vi "RT_Aerodynamic_Force_in_DLR_Navigation_Reference_System_2 (SubVI).vi"(0 "Data":dbl[][](array[numeric]), 2 "input cluster 3":T4, 5 "i":i32, 7 "output cluster":T3, 9 "Rotation":T1, 11 "Vehicle Parameters":T2) -> (4 "FA":dbl[](array[numeric]), 15 "FA_b":dbl[](array[numeric]))   [LabVIEW 2017]
uses:
  <vilib>/Analysis/coordinate.llb/Euler Rotation Order.ctl
  <vilib>/Analysis/baseanly.llb/Real A x B.vi
  <vilib>/Analysis/Matrix/Numeric/Conversions/Array To Matrix - RA.vi
  <vilib>/Analysis/Matrix/Numeric/Conversions/Array To Matrix - RA2.vi
  <vilib>/Analysis/Matrix/Numeric/Conversions/Matrix To Array - RM.vi
  <vilib>/Analysis/NI_AALPro.lvlib
  <vilib>/Analysis/Matrix/NI_Matrix.lvlib
  <vilib>/Analysis/NI_AALBase.lvlib
panel:
  out "FAl":dbl[](array[numeric])
  out "FAy":dbl[](array[numeric])
  out "FAp":dbl[](array[numeric])
  out "FA_long":dbl
  out "FA_yaw":dbl
  out "FA_pitch":dbl
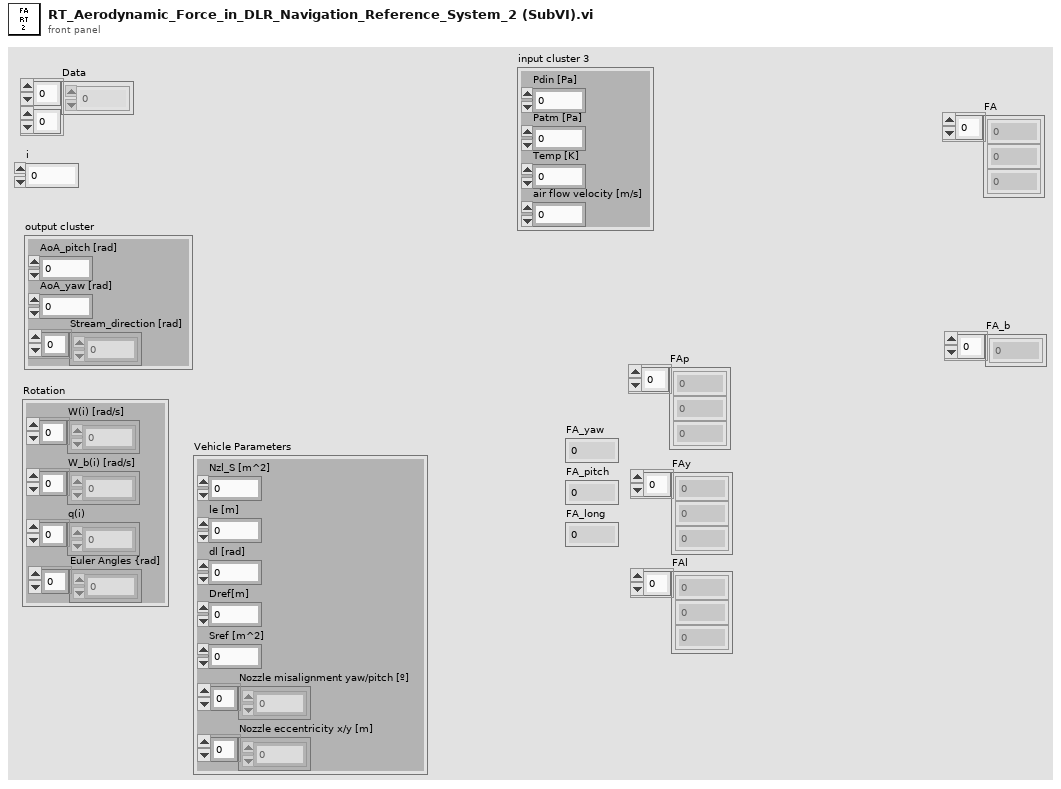
[diagram p1: front panel]
types:
  T1 = cluster{"W(i) [rad/s]":dbl[], "W_b(i) [rad/s]":dbl[], "q(i)":dbl[], "Euler Angles {rad]":dbl[]}
  T2 = cluster{"Nzl_S [m^2]":dbl, "le [m]":dbl, "dl [rad]":dbl, "Dref[m]":dbl, "Sref [m^2]":dbl, "Nozzle misalignment yaw/pitch [º]":dbl[], "Nozzle eccentricity x/y [m]":dbl[]}
  T3 = cluster{"AoA_pitch [rad]":dbl, "AoA_yaw [rad]":dbl, "Stream_direction [rad]":dbl[]}
  T4 = cluster{"Pdin [Pa]":dbl, "Patm [Pa]":dbl, "Temp [K]":dbl, "air flow velocity [m/s]":dbl}
  T5 = typedef "NI_AALPro.lvlib/Euler Rotation Order.ctl" = u16
  T6 = typedef "NI_Matrix.lvlib/RealMatrix.ctl" = dbl[][]
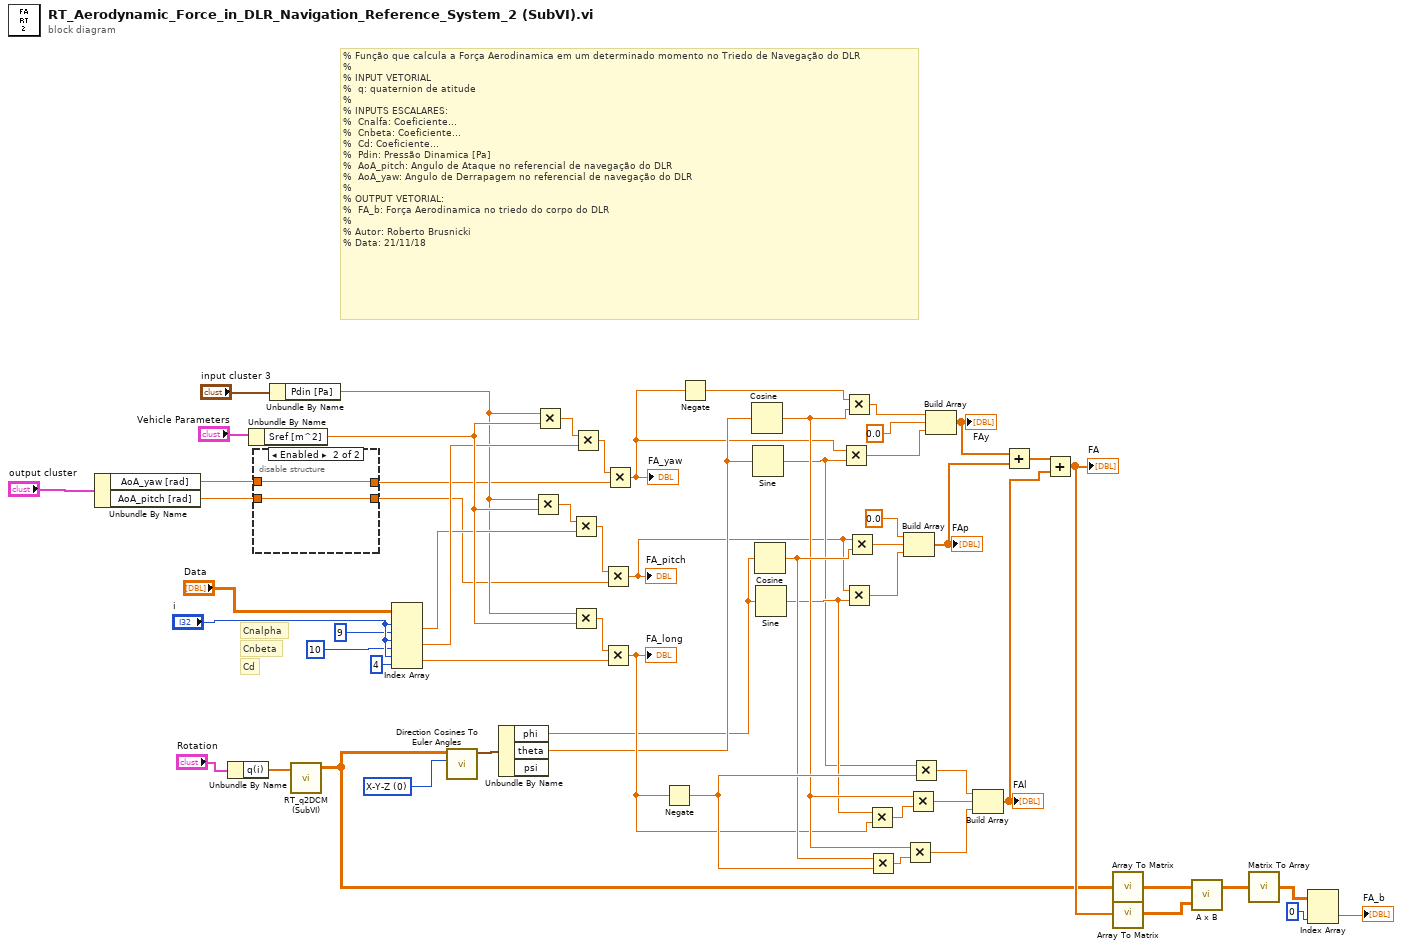
[diagram p0: block diagram]
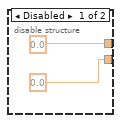
[diagram p2: hidden frame]
diagram:
  w24 = T5 0 items=["X-Y-Z", "X-Z-Y", "Y-X-Z", "Y-Z-X", "Z-X-Y", "Z-Y-X", "X-Y-X", "X-Z-X", "Y-X-Y", "Y-Z-Y", "Z-X-Z", "Z-Y-Z"] ("rotation order")
  # "% Função que calcula a Força Aerodinamica em um determinado momento no Triedo de Navegação do DLR\n%\n% INPUT VETORIAL\n%  q: quaternion de atitude\n%\n% INPUTS ESCALARES:\n%  Cnalfa: Coeficiente...\n%  Cnbeta: Coeficiente...\n%  Cd: Coeficiente...\n%  Pdin: Pressão Dinamica [Pa]\n%  AoA_pitch: Angulo de Ataque no referencial de navegação do DLR\n%  AoA_yaw: Angulo de Derrapagem no referencial de navegação do DLR\n%\n% OUTPUT VETORIAL:\n%  FA_b: Força Aerodinamica no triedo do corpo do DLR\n%\n% Autor: Roberto Brusnicki\n% Data: 21/11/18"
  # "Cd"
  # "Cnbeta"
  # "Cnalpha"
  n1 = Unbundle By Name("output cluster") -> ("AoA_yaw [rad]"=w11:dbl, "AoA_pitch [rad]"=w10:dbl)
  n2 = Unbundle By Name("Rotation") -> ("q(i)"=w5:dbl[])
  n3 = Unbundle By Name("Vehicle Parameters") -> ("Sref [m^2]"=w32:dbl)
  n4 = disable-structure shown="Enabled" {
    disable-tunnel: w11 -> [_ w64]
    disable-tunnel: w10 -> [_ w63]
    disable-tunnel: [0.0 ("AoA_pitch [rad]") w63] -> w2
    disable-tunnel: [0.0 ("AoA_yaw [rad]") w64] -> w1
    frame Disabled {
    }
    frame Enabled {
    }
  }
  n5 = Unbundle By Name("input cluster 3") -> ("Pdin [Pa]"=w9:dbl)
  n6 = call "RT_q2DCM (SubVI).vi"("Quaternion"=w5) -> ("DCM"=w4:dbl[][])  [unwired: 10 in]
  n7 = Index Array(array="Data", index (row) #1="i", index (col) #1=9 ("disabled index (col)"), index (row) #2="i", index (col) #2=10 ("disabled index (col)"), index (row) #3="i", index (col) #3=4 ("disabled index (col)")) -> (element #1=w25:dbl, element #2=w30:dbl, element #3=w33:dbl)
  n8 = call <vilib>:"Direction Cosines To Euler Angles.vi"("rotation order"=w24, "Direction Cosines"=w4) -> ("Euler Angles"=w34:cluster{"phi":dbl, "theta":dbl, "psi":dbl})  [unwired: 8 in, 1 out]
  n9 = Unbundle By Name(w34) -> ("phi"=w36:dbl, "theta"=w42:dbl)  [unwired: 1 out]
  n10 = Multiply(x=w9, y=w32) -> (x*y=w26:dbl)
  n11 = Multiply(x=w9, y=w32) -> (x*y=w29:dbl)
  n12 = Multiply(x=w26, y=w25) -> (x*y=w27:dbl)
  n13 = Multiply(x=w9, y=w32) -> (x*y=w31:dbl)
  n14 = Multiply(x=w29, y=w30) -> (x*y=w28:dbl)
  n15 = Multiply(x=w27, y=w2) -> (x*y=w35:dbl)
  "FA_pitch" <- w35
  n16 = Multiply(x=w31, y=w33) -> (x*y=w52:dbl)
  "FA_long" <- w52
  n17 = Multiply(x=w28, y=w1) -> (x*y=w40:dbl)
  "FA_yaw" <- w40
  n18 = Negate(x=w52) -> (-x=w56:dbl)
  n19 = Negate(x=w40) -> (-x=w41:dbl)
  n20 = Cosine(x=w42) -> (cos(x)=w53:dbl)
  n21 = Sine(x=w42) -> (sin(x)=w49:dbl)
  n22 = Cosine(x=w36) -> (cos(x)=w55:dbl)
  n23 = Sine(x=w36) -> (sin(x)=w51:dbl)
  n24 = Multiply(x=w40, y=w49) -> (x*y=w44:dbl)
  n25 = Multiply(x=w41, y=w53) -> (x*y=w43:dbl)
  n26 = Multiply(x=w35, y=w51) -> (x*y=w37:dbl)
  n27 = Multiply(x=w35, y=w55) -> (x*y=w38:dbl)
  n28 = Multiply(x=w51, y=w52) -> (x*y=w50:dbl)
  n29 = Multiply(x=w55, y=w56) -> (x*y=w54:dbl)
  n30 = Build Array(0.0 ("element"), w38, w37) -> (w58:dbl[])
  "FAp" <- w58
  n31 = Multiply(x=w53, y=w54) -> (x*y=w46:dbl)
  n32 = Multiply(x=w53, y=w50) -> (x*y=w47:dbl)
  n33 = Multiply(x=w49, y=w56) -> (x*y=w48:dbl)
  n34 = Build Array(w43, 0.0 ("element"), w44) -> (w57:dbl[])
  "FAy" <- w57
  n35 = Build Array(w48, w47, w46) -> (w60:dbl[])
  "FAl" <- w60
  n36 = Add(x=w57, y=w58) -> (x+y=w59:dbl[])
  n37 = Add(x=w59, y=w60) -> (x+y=w13:dbl[])
  "FA" <- w13
  n38 = call-poly <vilib>:"Array To Matrix.vi"("Real 2D Array"=w4) -> ("Real Matrix"=w14:T6)
  n39 = call-poly <vilib>:"Array To Matrix.vi"("Real 1D Array"=w13) -> ("Real Matrix (Column Vector)"=w17:T6)
  n40 = call-poly <vilib>:"A x B.vi"("B"=w17, "A"=w14) -> ("A x B"=w16:T6)  [unwired: 1 out]
  n41 = call-poly <vilib>:"Matrix To Array.vi"("Real Matrix"=w16) -> ("Real 2D Array"=w18:dbl[][])
  n42 = Index Array(array=w18, index (col)=0 ("index (row)")) -> (element=→"FA_b":dbl[])  [unwired: 1 in]
